vi "Get URI.vi"(11 "Register JSON in":refnum<class "Register JSON.lvclass">) -> (2 "URI":string, 3 "Register JSON out":refnum<class "Register JSON.lvclass">)   [LabVIEW 2020, in "wamplv.lvlib" / "Register JSON.lvclass"]
uses:
  Register JSON.lvclass
  Register JSON.lvclass/Register JSON.ctl
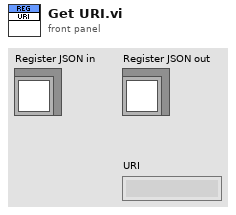
[diagram p1: front panel]
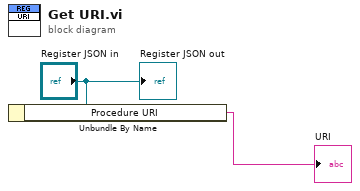
[diagram p0: block diagram]
diagram:
  n1 = Unbundle By Name("Register JSON in") -> ("Procedure URI"=→"URI":string)
  "Register JSON out" <- "Register JSON in"
